vi "Example Handler.vi"   [LabVIEW 2023]
uses:
  a08edaa9-a031-49df-9f8f-21c9c41081c9.vi
  <extravilib>/ChannelInstances/Messenger-t'Message Queue.lvlib-Message Cluster.ctl'.lvlib
  12c4b02a-eb75-4695-bdb9-7946f90e179e.vi
  Example Handler Clases.ctl
  <vilib>/Utility/error.llb/Error Cluster From Error Code.vi
  <vilib>/ErrorRing/Error Ring.xnode
  ee604d09-2f32-401b-854b-317be057be24.vi
  6096788f-46ba-4afd-b44e-2b7d8a4faf2e.vi
types:
  T1 = typedef "Example Handler Clases.ctl" = enum16{"Default", "Error", "Close", "Stop Module", "DoWork1"}
  T2 = typedef "Message Queue.lvlib/Message Cluster.ctl" = cluster{"Message":string, "Message Data":variant}
  T3 = typedef "Messenger-t'Message Queue.lvlib-Message Cluster.ctl'.lvlib/))Channel.ctl" = refnum<queue>
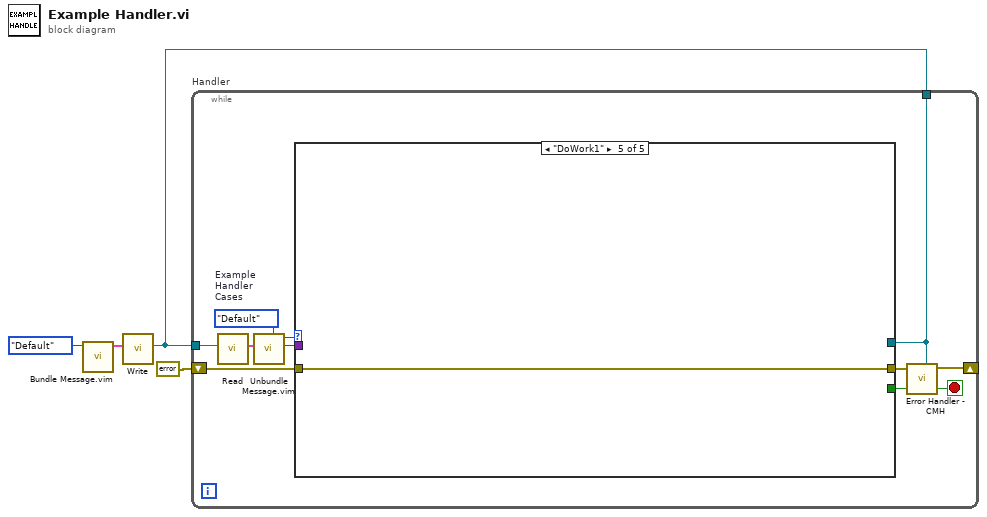
[diagram p0: block diagram]
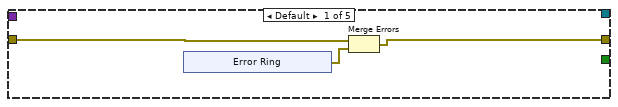
[diagram p2: hidden frame]
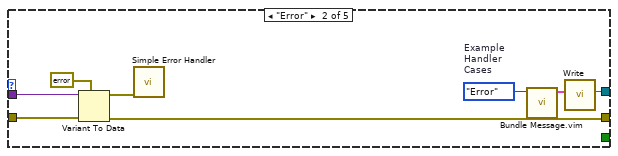
[diagram p3: hidden frame]
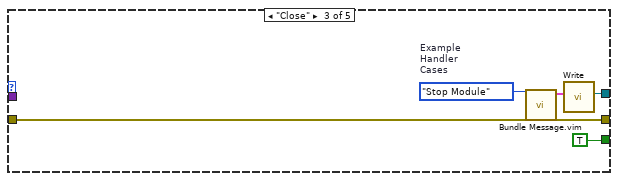
[diagram p4: hidden frame]
diagram:
  n1 = call "Bundle Message.vim"("Message"=Example_Handler_Clases."Default") -> ("Message Cluster"=w3:T2)  [unwired: 10 in]
  n2 = call <extravilib>:"Write.vi"("element"=w3) -> ("channel"=w1:T3)  [unwired: 8 in, 2 out]
  n3 = while "Handler" {
    tunnel: w1 -> [w14]
    shift-right: [w7] -> _
    shift-left: errorcluster {"status"=FALSE, "code"=0, "source"=""} ("error constant") -> [w9]
    tunnel: w1 -> [w5]
    stop <- w6 stop-if-true
    w11 = Example_Handler_Clases."Default"  # Example Handler Cases
    n4 = call <extravilib>:"Read.vi"("channel"=w14) -> ("element"=w13:T2)  [unwired: 8 in, 2 out]
    n5 = call "Unbundle Message.vim"("Case Type"=w11, "Message Cluster"=w13) -> ("Message Data"=w10:variant, "Message"=w12:T1)  [unwired: 8 in]
    n6 = case shown="\"DoWork1\"" w12 {
      tunnel: w10 -> [_ w27 _ _ _]
      tunnel: w9 -> [w16 w28 w35 w36 w37]
      tunnel: [w15 w26 w35 w36 w37] -> w8
      tunnel: [_ _ TRUE _ _] -> w6
      tunnel: [_ w23 w33 _ _] -> w5
      frame Default {
        n7 = xnode "Error Ring"() -> ("error out"=w17:errorcluster)
        n8 = Merge Errors(w16, w17) -> (w15:errorcluster)
      }
      frame "Error" {
        w25 = Example_Handler_Clases."Error"  # Example Handler Cases
        n9 = Variant To Data(error in=w28, type=errorcluster {"status"=FALSE, "code"=0, "source"=""} ("error in (no error)"), Variant=w27) -> (data=w29:errorcluster, error out=w26:errorcluster)
        n10 = call <vilib>:"Simple Error Handler.vi"("error in (no error)"=w29) -> ()  [unwired: 4 in, 5 out]
        n11 = call "Bundle Message.vim"("Message"=w25) -> ("Message Cluster"=w24:T2)  [unwired: 10 in]
        n12 = call <extravilib>:"Write.vi"("element"=w24) -> ("channel"=w23:T3)  [unwired: 8 in, 2 out]
      }
      frame "Close" {
        w32 = Example_Handler_Clases."Stop Module"  # Example Handler Cases
        n13 = call "Bundle Message.vim"("Message"=w32) -> ("Message Cluster"=w34:T2)  [unwired: 10 in]
        n14 = call <extravilib>:"Write.vi"("element"=w34) -> ("channel"=w33:T3)  [unwired: 8 in, 2 out]
      }
      frame "Stop Module" {
      }
      frame "DoWork1" {
      }
    }
    n15 = call "Error Handler - CMH.vi"("channel"=w5, "error in (no error)"=w8) -> ("error dup"=w7:errorcluster)  [unwired: 9 in]
  }
